vi "PH_Beckhoff_PP_PU.declare Sonderklemmen InputTags.vi"(0 "PU Type":T2) -> (1 "Description":string, 2 "Sonderklemmen Inputs":T3)   [LabVIEW 2014, in "PH_Beckhoff_PP_PU.lvlib"]
uses:
  PH_Beckhoff_PP_PU.lvlib
  PH_Beckhoff/PH_Beckhoff.Sonderklemmen Inputs.ctl
  PH_Beckhoff_PP_PU.PU Rack Type.ctl
  PH_Beckhoff_PP_PU.HV Meas Tags.ctl
  PH_Beckhoff/PH_Beckhoff.lvlib
panel:
  in  "Input Value":T1
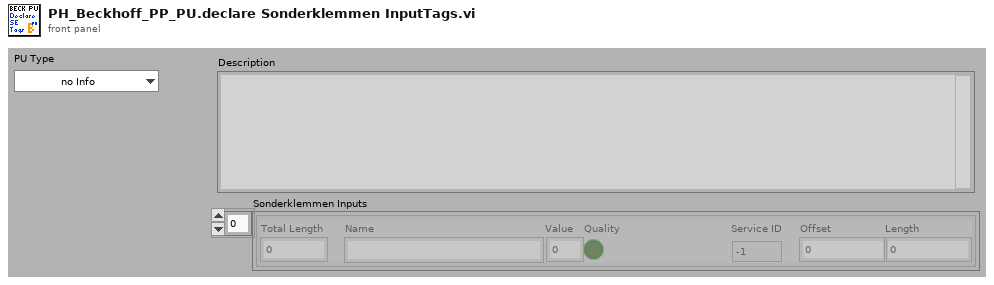
[diagram p1: front panel]
types:
  T1 = cluster{"Total Length":u32, "Name":string, "Value":u32, "Quality":bool, "Service ID":i32, "Offset":u32, "Length":u32}
  T2 = typedef "PH_Beckhoff_PP_PU.lvlib/PH_Beckhoff_PP_PU.PU Rack Type.ctl" = enum16{"no Info", "PA 19mm", "PA 45mm", "MA PU 1 and 2", "MA PU 3 and 4", "MA PU 5 and 6", "MA FR and PILC"}
  T3 = typedef "PH_Beckhoff.lvlib/PH_Beckhoff.Sonderklemmen Inputs.ctl" = cluster{"Total Length":u32, "Name":string, "Value":u64, "Quality":bool, "Service ID":i32, "Offset":u32, "Length":u32}[]
  T4 = typedef "PH_Beckhoff_PP_PU.lvlib/PH_Beckhoff_PP_PU.HV Meas Tags.ctl" = enum16{"voltage-raw", "voltage"}
  T5 = typedef "PH_PP_Common.lvlib/PH_PP_Common.PUs.ctl" = enum16{"no Info", "PA-19mm-1", "PA-19mm-2", "PA-45mm-PILC", "PA-45mm-MAIN", "MA-PU-1", "MA-PU-2", "MA-PU-3", "MA-PU-4", "MA-PU-5", "MA-PU-6", "MA-FR", "MA-PILC", "PA-45mm-DP"}
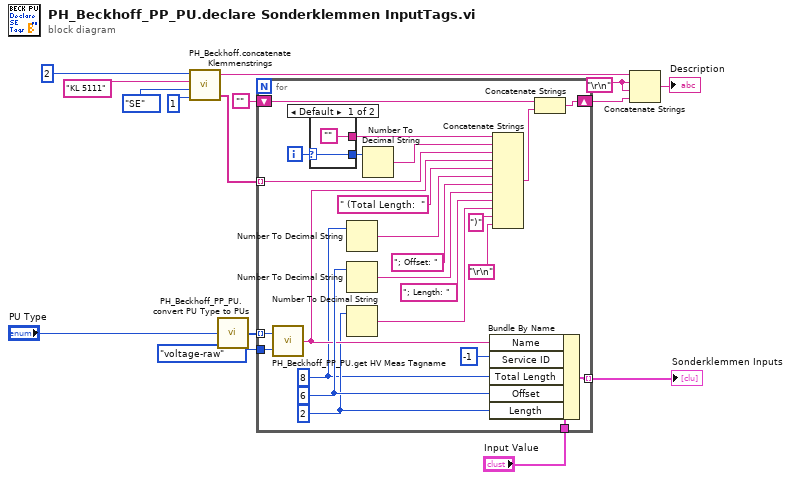
[diagram p0: block diagram]
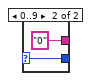
[diagram p2: hidden frame]
diagram:
  w13 = "\r\n"
  n1 = call "PH_Beckhoff.concatenate Klemmenstrings.vi"("# of In- or Outputs"=1, "Type"=enum16{"AE", "AA", "DE", "DA", "SE"}."SE", "Klemmenname"="KL 5111", "Quantity"=2) -> ("concatenated string array"=w7:string[], "\"<Type>: <Quantity> x <Klemmenname>\""=w8:string)  [unwired: 1 out]
  n2 = call "PH_Beckhoff_PP_PU.convert PU Type to PUs.vi"("PU Type"="PU Type") -> ("PUs"=w1:T5[])
  n3 = for {
    tunnel: w7 -> [w36] mode=indexing
    shift-right: [w33] -> w14
    shift-left: "" -> [w32]
    tunnel: "Input Value" -> [w30]
    tunnel: [w29] -> w5 mode=indexing
    tunnel: PH_Beckhoff_PP_PU.HV_Meas_Tags."voltage-raw" ("HV Meas Tag") -> [w24]
    tunnel: w1 -> [w23] mode=indexing
    i -> [w40]
    w19 = u32 2 ("Length")
    w16 = u32 8 ("Length")
    w28 = u32 6 ("Offset")
    n4 = call "PH_Beckhoff_PP_PU.get HV Meas Tagname.vi"("HV Meas Tag"=w24, "PU"=w23) -> ("HV Meas Tagname"=w25:string)
    n5 = case shown="Default" w40 {
      selector: w40 -> [w41 w44]
      tunnel: [w41 w44] -> w39
      tunnel: ["" "0"] -> w38
      frame Default {
      }
      frame 0..9 {
      }
    }
    n6 = Number To Decimal String(number=w16) -> (decimal integer string=w17:string)  [unwired: 1 in]
    n7 = Number To Decimal String(number=w28) -> (decimal integer string=w22:string)  [unwired: 1 in]
    n8 = Number To Decimal String(number=w19) -> (decimal integer string=w20:string)  [unwired: 1 in]
    n9 = Number To Decimal String(number=w39) -> (decimal integer string=w37:string)  [unwired: 1 in]
    n10 = Bundle By Name(cluster=w30, "Name"=w25, "Service ID"=-1, "Total Length"=w16, "Offset"=w28, "Length"=w19) -> (w29:T1)
    n11 = Concatenate Strings(w38, w37, w36, w25, " (Total Length:  " ("string"), w17, "; Offset: " ("string"), w22, "; Length: " ("string"), w20, ")" ("string"), "\r\n") -> (w34:string)
    n12 = Concatenate Strings(w32, w34) -> (w33:string)
  }
  "Sonderklemmen Inputs" <- w5
  n13 = Concatenate Strings(w8, w13, w13, w14) -> (→"Description":string)
